vi "NI VeriStand - Signal When Ready for Shutdown.vi"(8 "error in (no error)":errorcluster) -> (0 "error out":errorcluster)   [LabVIEW 2020, in "Custom Device API.lvlib"]
doc: "Signals that the <B>System Explorer</B> window is ready to go into idle mode. Ensure all changes are saved before calling this VI."
uses:
  <vilib>/NI VeriStand/Custom Device API/Custom Device API.lvlib
  65951b20-b0d6-4088-b73d-dd65903e175e.vi
  <vilib>/NI VeriStand/Custom Device API/Custom Device Offline Path.vi
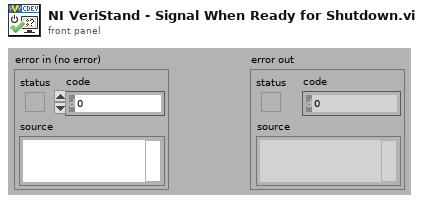
[diagram p1: front panel]
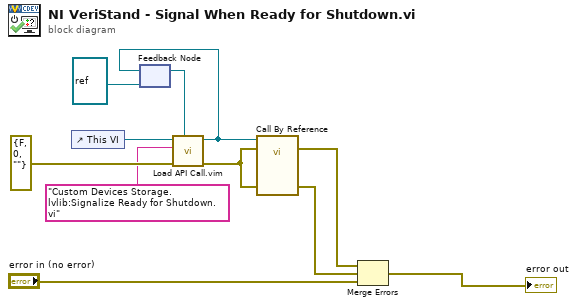
[diagram p0: block diagram]
diagram:
  n1 = control-ref of="This VI"() -> (w7:refnum<vi>)
  n2 = feedback #1(refnum<vi> refnum ("type specifier VI Refnum (for type only)")) -> (w8:refnum<vi>)
  n3 = call "Load API Call.vim"("VI reference in"=w8, "error in (no error)"=errorcluster {"status"=FALSE, "code"=0, "source"=""}, "VI qualified name"="Custom Devices Storage.lvlib:Signalize Ready for Shutdown.vi", "Caller VI ref"=w7) -> ("error out"=w3:errorcluster, "VI reference"=w6:refnum<vi>)  [unwired: 6 in]
  n4 = feedback-in #1(w6) -> ()
  n5 = call-by-ref "?"(reference=w6, error in=w3, 8:"error in (no error)"=w3) -> (error out=w1:errorcluster, 0:"error out"=w11:errorcluster)  [unwired: 10 in, 1 out]
  n6 = Merge Errors(w1, w11, "error in (no error)") -> (→"error out":errorcluster)
